vi "move.vi"() -> ()   [LabVIEW 2017]
doc: "This uses an event structure with a \"Mouse Move\" event to track the position of the mouse and adjust the coordinates of the control/indicator accordingly. This adjustment only occurs when the mouse has been clicked on the control/indicator."
uses:
  <vilib>/Utility/miscctls.llb/LVBoundsTypeDef.ctl
panel:
  in  "reference":refnum<vi>
  out "Cluster":T1
  in  "stop":bool
  # "Overview: In this VI the front panel control/indicator is moved while the mouse is moving and not after the mouse button has been released.\n\nRequirements: LabVIEW 2012 (or compatible).\n\nInstructions:\n1. Run the VI.\n2. Click on the Boolean control.\n3. Move the mouse.\n4. Release mouse.\n5. Stop the VI."
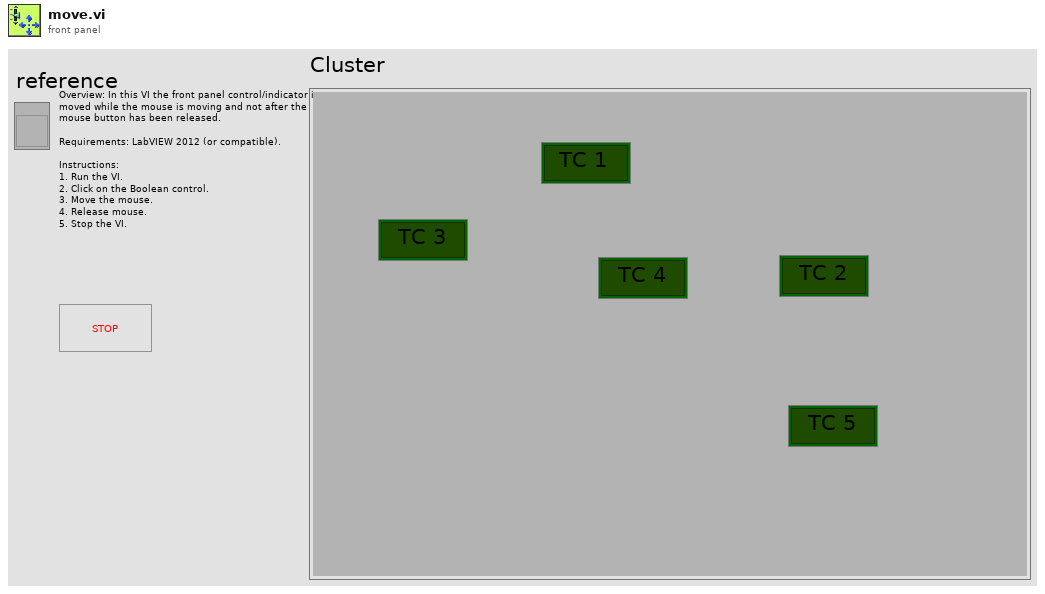
[diagram p1: front panel]
types:
  T1 = cluster{"TC 1":bool, "TC 2":bool, "TC 3":bool, "TC 4":bool, "TC 5":bool}
  T2 = typedef "LVBoundsTypeDef.ctl" = cluster{"Width":u32, "Height":u32}
  T3 = typedef "LVPoint32TypeDef.ctl" = cluster{"Horizontal":i32, "Vertical":i32}
  T4 = typedef "LVPositionTypeDef.ctl" = cluster{"Left":i32, "Top":i32}
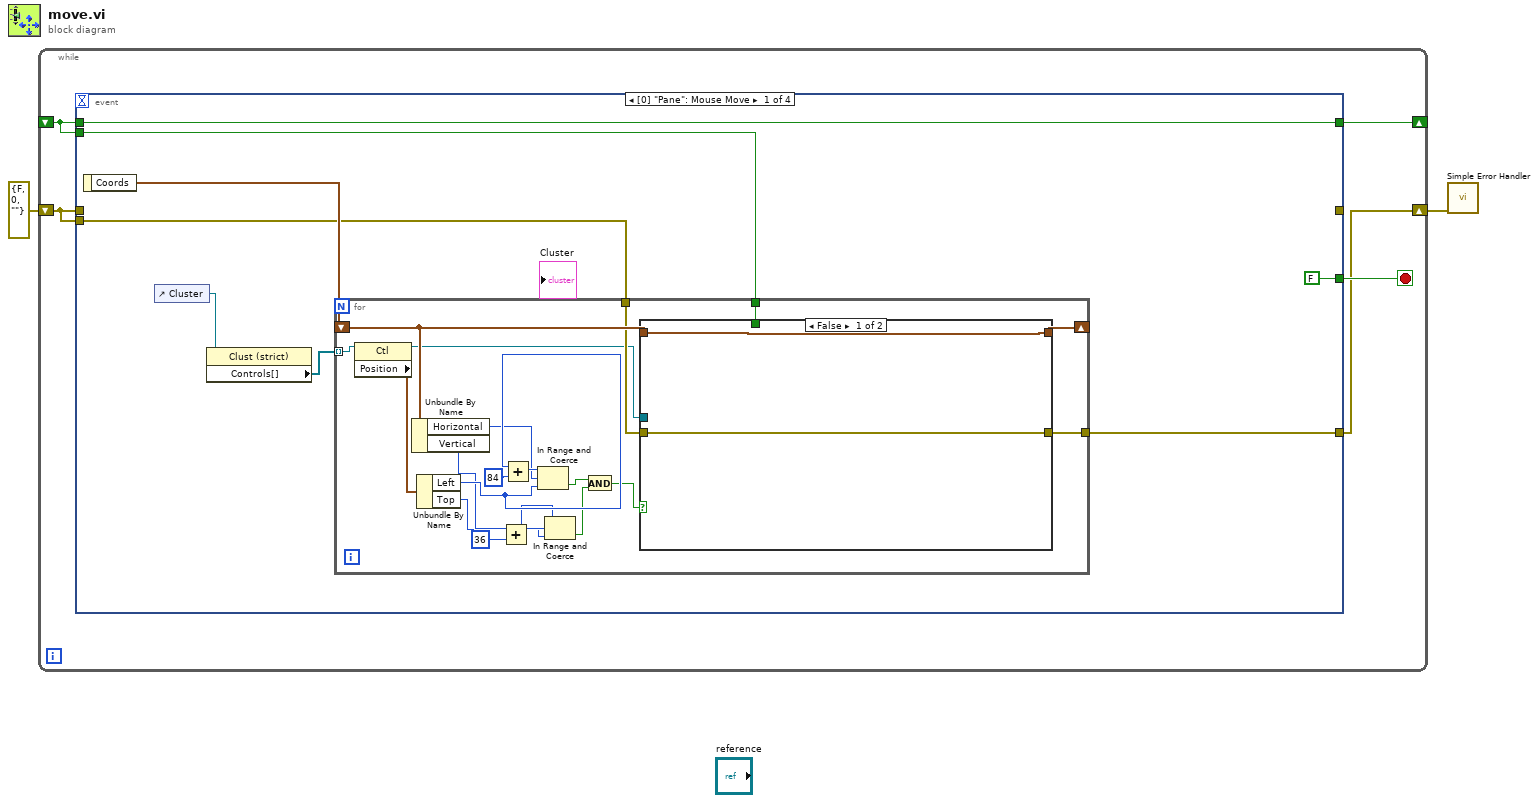
[diagram p0: block diagram]
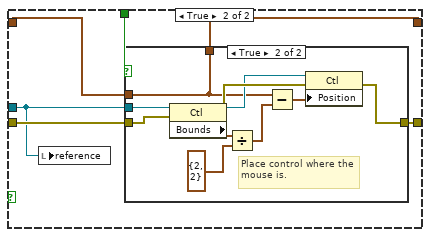
[diagram p2: hidden frame]
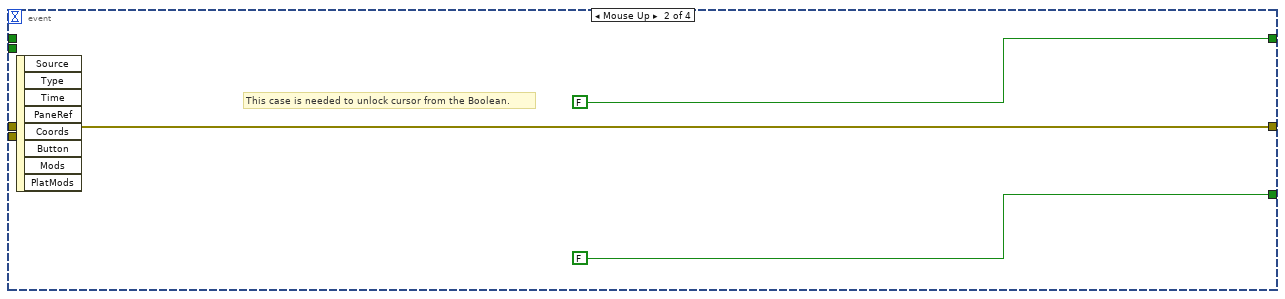
[diagram p4: hidden frame]
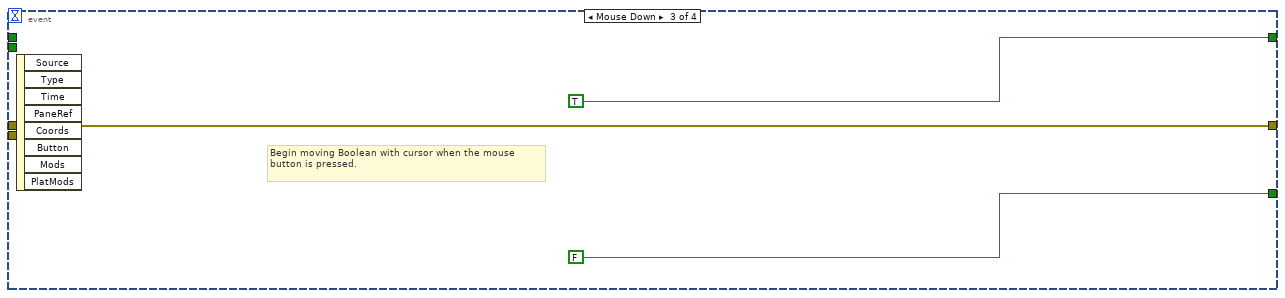
[diagram p5: hidden frame]
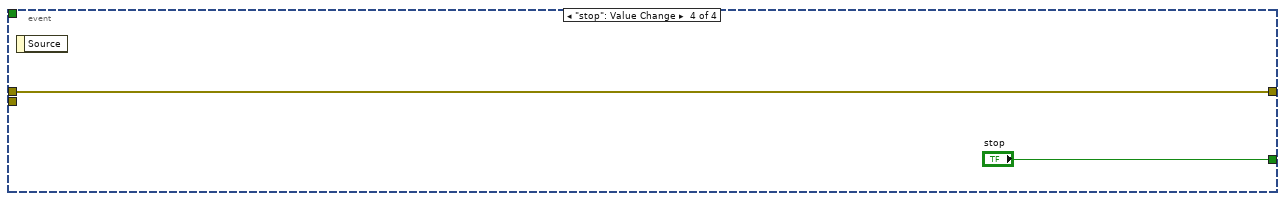
[diagram p6: hidden frame]
diagram:
  n1 = while {
    shift-right: [w6] -> _
    shift-left: _ -> [w5]
    shift-right: [w3] -> w1
    shift-left: errorcluster {"status"=FALSE, "code"=0, "source"=""} ("error out") -> [w4]
    stop <- w7 stop-if-true
    n2 = event shown="[0] \"Pane\": Mouse Move" {
      selector: _ -> [_ _ _ _]
      dyn-events: _ -> [_ _ _ _]
      timeout: _ -> [_ _ _ _]
      tunnel: [FALSE ("stop") FALSE ("stop") FALSE ("stop") "stop"] -> w7
      tunnel: [w15 FALSE TRUE _] -> w6
      tunnel: w5 -> [w15 _ _ _]
      tunnel: w4 -> [_ w55 w58 w61]
      tunnel: [_ w55 w58 w61] -> _
      tunnel: w5 -> [w10 _ _ _]
      tunnel: w4 -> [w9 _ _ _]
      tunnel: [w8 _ _ _] -> w3
      event Mouse Move {
        n3 = event-data() -> ("Coords"=w11:T3)  [unwired: 1 out]
        n4 = control-ref of="Cluster"() -> (w13:refnum<vi>)
        n5 = property class="Clust (strict)"(reference=w13) -> ("Controls[]"=w12:refnum<vi>[])  [unwired: 1 in, 2 out]
        n6 = for {
          tunnel: w12 -> [w25] mode=indexing
          shift-right: [w20] -> _
          shift-left: w11 -> [w24]
          tunnel: w10 -> [w23]
          tunnel: w9 -> [w22]
          tunnel: [w21] -> w8
          n7 = property on="Property Node" class="Ctl"(reference=w25) -> (reference out=w19:refnum<vi>, "Position"=w34:T4)  [unwired: 1 in, 1 out]
          n8 = Unbundle By Name(w24) -> ("Horizontal"=w29:i32, "Vertical"=w28:i32)
          n9 = Unbundle By Name(w34) -> ("Left"=w30:i32, "Top"=w26:i32)
          n10 = Add(x=w26, y=36) -> (x+y=w27:i32)
          n11 = Add(x=w30, y=84) -> (x+y=w33:i32)
          n12 = In Range and Coerce(upper limit=w33, x=w29, lower limit=w30) -> (In Range?=w18:bool)  [unwired: 1 out]
          n13 = In Range and Coerce(upper limit=w27, x=w28, lower limit=w26) -> (In Range?=w17:bool)  [unwired: 1 out]
          n14 = And(x=w18, y=w17) -> (x .and. y?=w16:bool)
          n15 = case shown="False" w16 {
            tunnel: w24 -> [w36 w42]
            tunnel: w23 -> [_ w41]
            tunnel: w22 -> [w35 w40]
            tunnel: [w35 w39] -> w21
            tunnel: [w36 w38] -> w20
            tunnel: w19 -> [_ w37]
            frame False {
            }
            frame True {
              n16 = local write "reference"(w37) -> ()
              n17 = case shown="True" w41 {
                tunnel: w42 -> [w43 w46]
                tunnel: w40 -> [w44 w50]
                tunnel: [w44 w48] -> w39
                tunnel: w37 -> [_ w45]
                tunnel: [w43 w46] -> w38
                frame False {
                }
                frame True {
                  # "Place control where the mouse is."
                  n18 = property on="Property Node" class="Ctl"(reference=w45, error in=w50) -> (reference out=w47:refnum<vi>, error out=w49:errorcluster, "Bounds"=w54:T2)
                  n19 = Divide(x=w54, y=T2 {"Width"=2, "Height"=2}) -> (x/y=w52:cluster{"Width":dbl, "Height":dbl})
                  n20 = Subtract(x=w46, y=w52) -> (x-y=w53:cluster{dbl, dbl})
                  n21 = property on="Property Node" class="Ctl"(reference=w47, error in=w49, "Position"=w53) -> (error out=w48:errorcluster)  [unwired: 1 out]
                }
              }
            }
          }
        }
      }
      event Mouse Up {
        # "This case is needed to unlock cursor from the Boolean."
        n22 = event-data() -> ()  [unwired: 9 out]
      }
      event Mouse Down {
        # "Begin moving Boolean with cursor when the mouse button is pressed."
        n23 = event-data() -> ()  [unwired: 9 out]
      }
      event "stop": Value Change {
        n24 = event-data() -> ()  [unwired: 2 out]
      }
    }
  }
  n25 = call <vilib>:"Simple Error Handler.vi"("error in (no error)"=w1) -> ()  [unwired: 4 in, 5 out]
